vi "Run.vi"(8 "error in (no error)":errorcluster, 11 "RoomAlert in":refnum<class "RoomAlert.lvclass">) -> (0 "error out":errorcluster, 1 "DataValid":bool, 2 "clSensorData":T1, 3 "RoomAlert out":refnum<class "RoomAlert.lvclass">)   [LabVIEW 2018, in "SensorPlugins.lvlib" / "RoomAlert.lvclass"]
doc: "Retrieves measurements from the RoomAlert instrument."
uses:
  RoomAlert.lvclass
  SensorShared/clSensorData.ctl
  SensorShared/SensorVisulization.ctl
  <vilib>/Utility/error.llb/Error Cluster From Error Code.vi
  <vilib>/ErrorRing/Error Ring.xnode
  SensorShared/SensorShared.lvlib
panel:
  out "Execution Time (ms)":u32
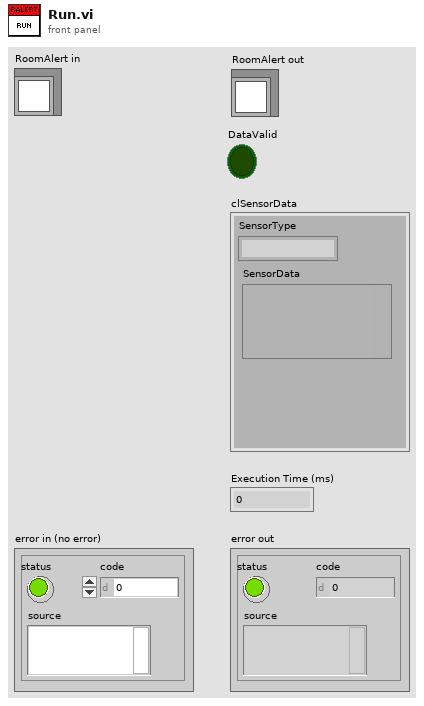
[diagram p1: front panel]
types:
  T1 = typedef "SensorShared.lvlib/clSensorData.ctl" = cluster{"SensorType":string, "SensorData":variant}
  T2 = typedef "SensorShared.lvlib/SensorVisulization.ctl" = cluster{"Array of Waveforms":waveform(dbl)[], "Array of Strings ":string[], "LightTower":cluster{"Red":bool, "Amber":bool, "Green":bool, "Audio":bool}}
  T3 = typedef "SensorPlugins.lvlib/RoomAlert.lvclass/RoomAlertControls.ctl" = cluster{"Connected?":bool, "IP Address of SNMP Device":string, "Port (161)":u16, "Community Name":string, "Measurements To Read Array":u16[], "Update LightTower?":bool, "LightTower":cluster{"Red":bool, "Amber":bool, "Green":bool, "Audio":bool}, "RoomAlert Model ID":string, "Sensor OID Numbers":string[][], "Sensor Light Tower OID Numbers":string[][]}[]
  T4 = typedef "SensorPlugins.lvlib/RoomAlert.lvclass/CommunicationControls.ctl" = refnum<k16>[]
  T5 = typedef "SensorPlugins.lvlib/RoomAlert.lvclass/MeasurementControls.ctl" = cluster{"Measurement RefreshTime (ms)":u32, "Measurement Name":string, "Timeout(ms)":i32, "Amber Warning Light Configuration":cluster{"Warning Temperture (Degrees C)":dbl, "Temperature Delta (Degrees C/Minute)":dbl, "Time Window (Minutes)":dbl}}
  T6 = cluster{"Warning Temperture (Degrees C)":dbl, "Temperature Delta (Degrees C/Minute)":dbl, "Time Window (Minutes)":dbl}
  T7 = cluster{"[0]":bool, "[1]":bool, "[2]":bool, "[3]":bool}
  T8 = cluster{"Connected?":bool, "IP Address of SNMP Device":string, "Port (161)":u16, "Community Name":string, "Measurements To Read Array":u16[], "Update LightTower?":bool, "LightTower":cluster{"Red":bool, "Amber":bool, "Green":bool, "Audio":bool}, "RoomAlert Model ID":string, "Sensor OID Numbers":string[][], "Sensor Light Tower OID Numbers":string[][]}
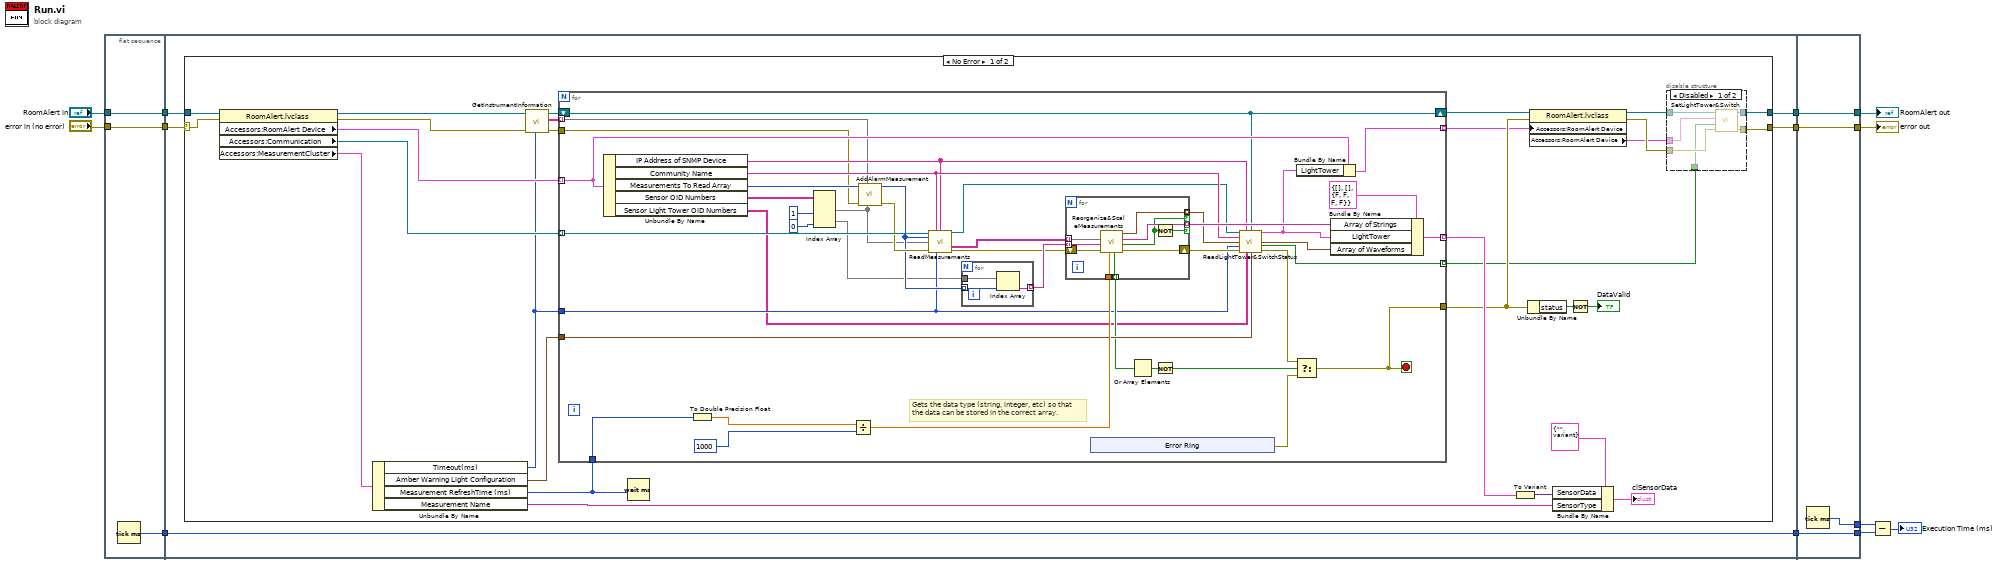
[diagram p0: block diagram]
diagram:
  n1 = flat-sequence {
    tunnel: "RoomAlert in" -> [w15]
    tunnel: "error in (no error)" -> [w16]
    tunnel: [w16] -> w13
    tunnel: [w15] -> w12
    tunnel: [w14] -> w11
    tunnel: w13 -> [w21]
    tunnel: w12 -> [w20]
    tunnel: [w19] -> w8
    tunnel: [w18] -> w9
    tunnel: w11 -> [w17]
    tunnel: [w17] -> w10
    tunnel: [w122] -> w4
    tunnel: [w123] -> w5
    tunnel: w10 -> [w120]
    tunnel: w9 -> [w122]
    tunnel: w8 -> [w123]
    tunnel: [w121] -> w2
    tunnel: [w120] -> w1
    frame #0 {
      n2 = Tick Count (ms)() -> (millisecond timer value=w14:u32)
    }
    frame #1 {
      n3 = case shown="No Error" w21 {
        selector: w21 -> [w49 w119]
        tunnel: w20 -> [w50 w118]
        tunnel: [w36 w119] -> w18
        tunnel: [w34 w118] -> w19
        frame No Error {
          n4 = property class="RoomAlert.lvclass"(reference=w50, error in=w49) -> (reference out=w30:refnum<class "RoomAlert.lvclass">, error out=w28:errorcluster, "Accessors:RoomAlert Device"=w46:T3, "Accessors:Communication "=w41:T4, "Accessors:MeasurementCluster"=w40:T5)
          n5 = Unbundle By Name(w40) -> ("Timeout(ms)"=w23:i32, "Amber Warning Light Configuration"=w22:T6, "Measurement RefreshTime (ms)"=w24:u32, "Measurement Name"=w25:string)
          n6 = call "GetInstrumentInformation.vi"("Timeout(ms)"=w23, "error in (no error)"=w28, "RoomAlert in"=w30) -> ("error out"=w27:errorcluster, "Model IDs"=w26:string[][][], "RoomAlert out"=w29:refnum<class "RoomAlert.lvclass">)  [unwired: 6 in]
          n7 = for {
            tunnel: w46 -> [w64] mode=indexing
            tunnel: [w75] -> w38
            tunnel: [w91] -> w44 mode=indexing
            tunnel: w41 -> [w90] mode=indexing
            tunnel: w22 -> [w80]
            tunnel: [w73] -> w33 mode=indexing
            shift-right: [w60] -> w39
            shift-left: w29 -> [w60]
            tunnel: [w66] -> w31 mode=indexing
            tunnel: w27 -> [w57]
            tunnel: w26 -> [w61] mode=indexing
            tunnel: w23 -> [w59]
            tunnel: w24 -> [w58]
            stop <- w75 stop-if-true
            # "Gets the data type (string, integer, etc) so that\nthe data can be stored in the correct array."
            n8 = Unbundle By Name(w64) -> ("IP Address of SNMP Device"=w82:string, "Community Name"=w83:string, "Measurements To Read Array"=w65:u16[], "Sensor OID Numbers"=w56:string[][], "Sensor Light Tower OID Numbers"=w51:string[][])
            n9 = To Double Precision Float(number=w58) -> (double precision float=w88:dbl)
            n10 = Index Array(array=w56, index (col) #1=1 ("disabled index (col)"), index (col) #2=0 ("index (col)")) -> (element #1=w54:string[], element #2=w52:string[])  [unwired: 2 in]
            n11 = Divide(x=w88, y=u32 1000) -> (x/y=w86:dbl)
            n12 = call "AddAlarmMeasurement.vi"("OID Numbers"=w54, "Model Information"=w61, "Error In"=w57, "Measurements To Read Array In"=w65) -> ("Error Out"=w63:errorcluster, "Measurements To Read Array Out"=w62:u16[])  [unwired: 6 in]
            n13 = call "ReadMeasurements.vi"("UDP Network Connection in"=w90, "Community Name"=w83, "IP Address of SNMP Device"=w82, "Measurements To Read Array"=w62, "OID Numbers"=w54, "error in (no error)"=w63, "Timeout(ms)"=w59) -> ("UDP Network Connection out"=w69:refnum<k16>, "SNMPDataAsStrings"=w81:string[][], "error out"=w72:errorcluster)  [unwired: 6 in]
            n14 = for {
              tunnel: w62 -> [w98] mode=indexing
              tunnel: w52 -> [w99]
              tunnel: [w97] -> w84 mode=indexing
              n15 = Index Array(array=w99, index=w98) -> (element=w97:string)
            }
            n16 = for {
              tunnel: w81 -> [w100] mode=indexing
              shift-right: [w108] -> w71
              shift-left: w72 -> [w109]
              tunnel: [w107] -> w68 mode=indexing if=w104
              tunnel: w86 -> [w103]
              tunnel: [w106] -> w87 mode=indexing if=w105
              tunnel: w84 -> [w101] mode=indexing
              tunnel: [w102] -> w79 mode=indexing
              n17 = call "Reorganize&ScaleMeasurements.vi"("Meas Aperature"=w103, "Error In"=w109, "MeasurementType"=w101, "SNMPDataAsStrings"=w100) -> ("Error Out"=w108:errorcluster, "Numerical Information"=w104:bool, "String Data"=w106:string, "output waveform"=w107:waveform(dbl), "Alarmed"=w102:bool)  [unwired: 3 in]
              n18 = Not(x=w104) -> (.not. x?=w105:bool)
            }
            n19 = xnode "Error Ring"() -> ("error out"=w78:errorcluster)
            n20 = Or Array Elements(Boolean array=w79) -> (logical OR=w77:bool)
            n21 = Not(x=w77) -> (.not. x?=w76:bool)
            n22 = call "ReadLightTower&SwitchStatus.vi"("UDP Network Connection in"=w69, "IP Address of SNMP Device"=w82, "RoomAlert in"=w60, "Community Name"=w83, "Array In"=w68, "Timeout(ms)"=w59, "error in (no error)"=w71, "LightTower OID"=w51, "Amber Warning Light Limits"=w80) -> ("Light Tower"=w74:T7, "Array Out"=w67:waveform(dbl)[], "Yellow Limit Exceeded?"=w66:bool, "error out"=w70:errorcluster)  [unwired: 3 in]
            n23 = Select(t=w70, s=w76, f=w78) -> (s? t:f=w75:errorcluster)
            n24 = Bundle By Name(cluster=w64, "LightTower"=w74) -> (w73:T8)
            n25 = Bundle By Name(cluster=T2 {"Array of Waveforms"=[], "Array of Strings "=[], "LightTower"={"Red"=FALSE, "Amber"=FALSE, "Green"=FALSE, "Audio"=FALSE}} ("SiemensDEMMeasurements 2"), "Array of Strings"=w87, "LightTower"=w74, "Array of Waveforms"=w67) -> (w91:T2)
          }
          n26 = Wait (ms)(milliseconds to wait=w24) -> ()  [unwired: 1 out]
          n27 = To Variant(anything=w44) -> (Variant=w47:variant)
          n28 = Unbundle By Name(w38) -> ("status"=w45:bool)
          n29 = property class="RoomAlert.lvclass"(reference=w39, error in=w38, "Accessors:RoomAlert Device"=w33) -> (reference out=w35:refnum<class "RoomAlert.lvclass">, error out=w37:errorcluster, "Accessors:RoomAlert Device"=w32:T3)
          n30 = Bundle By Name(cluster=T1 {"SensorType"="", "SensorData"=variant} ("clSensorData"), "SensorData"=w47, "SensorType"=w25) -> (→"clSensorData":T1)
          n31 = Not(x=w45) -> (.not. x?=→"DataValid":bool)
          n32 = disable-structure shown="Disabled" {
            disable-tunnel: w37 -> [w115 w117]
            disable-tunnel: [w114 w117] -> w36
            disable-tunnel: w35 -> [w113 w116]
            disable-tunnel: [w112 w116] -> w34
            disable-tunnel: w32 -> [w111 _]
            disable-tunnel: w31 -> [w110 _]
            frame Disabled {
              n33 = call-dynamic "SetLightTower&Switch.vi"("error in (no error)"=w115, "UpdateValue? (F)"=w110, "RoomAlert Device"=w111, "RoomAlert in"=w113) -> ("error out"=w114:errorcluster, "RoomAlert out"=w112:refnum<class "RoomAlert.lvclass">)  [unwired: 6 in]
            }
            frame Enabled {
            }
          }
        }
        frame Error {
        }
      }
    }
    frame #2 {
      n34 = Tick Count (ms)() -> (millisecond timer value=w121:u32)
    }
  }
  n35 = Subtract(x=w2, y=w1) -> (x-y=→"Execution Time (ms)":u32)
  "error out" <- w4
  "RoomAlert out" <- w5
